vi "Write CorrectionFactors.vi"(8 "error in (no error)":errorcluster, 10 "CorrectionFactors":T1, 11 "SamplerPluginsBase in":refnum<class "SamplerPluginsBase.lvclass">) -> (0 "error out":errorcluster, 3 "SamplerPluginsBase out":refnum<class "SamplerPluginsBase.lvclass">)   [LabVIEW 2014, in "SamplerPlugins.lvlib" / "SamplerPluginsBase.lvclass"]
uses:
  SamplerPluginsBase.lvclass
  TypeDefs/CorrectionFactors.ctl
  SamplerPluginsBase.lvclass/SamplerPluginsBase.ctl
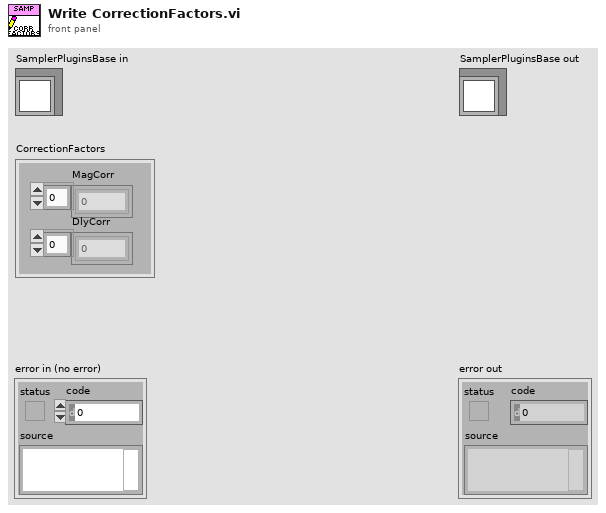
[diagram p1: front panel]
types:
  T1 = typedef "SamplerPlugins.lvlib/SamplerPluginsBase.lvclass/CorrectionFactors.ctl" = cluster{"MagCorr":dbl[], "DlyCorr":dbl[]}
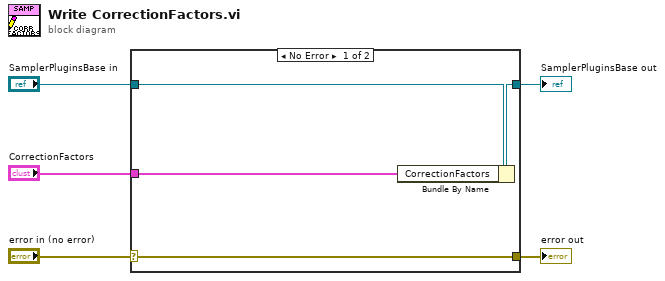
[diagram p0: block diagram]
diagram:
  n1 = case shown="No Error" "error in (no error)" {
    selector: "error in (no error)" -> [w9 w10]
    tunnel: [w9 w10] -> w4
    tunnel: [w7 w11] -> w2
    tunnel: "SamplerPluginsBase in" -> [w8 w11]
    tunnel: "CorrectionFactors" -> [w6 _]
    frame No Error {
      n2 = Bundle By Name(cluster=w8, "CorrectionFactors"=w6) -> (w7:refnum<class "SamplerPluginsBase.lvclass">)
    }
    frame Error {
    }
  }
  "error out" <- w4
  "SamplerPluginsBase out" <- w2
